vi "ProCoDA.vi"() -> ()   [LabVIEW 2015]
uses:
  Plant mode.ctl
  toolbar icons/open configuration.ctl
  toolbar icons/Save configuration.ctl
  toolbar icons/calibrator.ctl
  toolbar icons/edit rules.ctl
  switch and fraction.ctl
  toolbar icons/Data Source.ctl
  toolbar icons/file comment.ctl
  toolbar icons/log data.ctl
  TCP DAQ/Sensor data.ctl
  DAQ configuration/sensor cluster.ctl
  toolbar icons/peristaltic pump.ctl
  toolbar icons/help.ctl
  toolbar icons/Export pcm.ctl
  new config file.ctl
  calibration/Shared Data/share data boolean.ctl
  <vilib>/Utility/miscctls.llb/LVPositionTypeDef.ctl
  Plant state.ctl
  Distributed Daq/Data cmd.ctl
  DAQ configuration/Sensor buffer command.ctl
  file/file action.ctl
  Stamp/calibration commands.ctl
  default or user select.ctl
  calibration/Shared Data/share data command.ctl
  Calibration and Function folders.ctl
  <vilib>/Platform/browser.llb/Open URL in Default Browser (string).vi
panel:
  out "Legend:Position":T1
  in  "Swap Instance":T2
  in  "Name":string
  in  "Quit":bool
  out "auto datalogref":refnum<file>
  out "user datalog ref":refnum<file>
  in  "Tab Control":T3(tab)=enum."Process Operation"
  in  "Share data":T4
  in  "Datalog directory path":path
  in  "Auto data log interval":dbl=60.0 min=1.0 step=1.0
  out "Data Source":string
  in  "export pcm":T5
  out "sensor range error":bool
  out "Daq failure":bool
  in  "Peristaltic Pump":T6
  in  "Data Source":T7 caption="OK Button"
  out "data rate (Hz)":dbl
  out "Datalog File Failure":bool
  in  "Calibrate Sensors":T8
  in  "Edit Rules":T9
  in  "Save":T10
  in  "open":T11
  in  "Help Button":T12
  in  "File Comment":T13
  in  "Log Data":T14
  in  "User Data log interval":dbl=5.0 min=0.002 step=0.002
  out "read error":bool
  in  "Scrollbar":i32(c297)
  out "output descriptions":string[][](array[string])
  out "controls":T15 {"fractional duty" format="%#_3g"}
  in  "Operator Selected State":u16(ring)=1 items=["OFF", "Run pump"]
  out "Elapsed time in current state":dbl format="%.2f"
  out "Process State":u16(ring)=1 items=["OFF", "Run pump"]
  in  "Mode of Operation":T16=enum."Automatic Operation"
  out "Variables":cluster{string, "value":dbl}[](array[cluster]) {"value" format="%#_2g"}
  in  "history length":i32=1000 min=1
  in  "graph update interval":sgl=1.0 min=0.0001 format="%.4f"
  in  "Clear graph":bool
  out "Sensor Data":T17 {"Sensor array"."scaled" format="%.2f"; "Sensor array"."voltage" format="%.4f"; "Time" format="%<%I:%M:%S%2u %p\n%m/%d/%Y>T"}
  out "state graph":cluster{dbl[], dbl[]}(graph)
  in  "data to plot":i32[](listbox)
  out "Sensor graph":cluster{dbl[], dbl[]}[](graph)
  # "Method files (sensors, rules, calibrations)"
  # "Pump calibration"
  # "Calibrate the Analog Out"
  # "NI Input/Output device"
  # "Sensor configuration and calibration\nMeasure pH, D.O., Absorbance, etc."
  # "Data logging for experiments that span multiple days or if you need a state log."
  # "Control: states, rules, setpoints\nProgram the logic"
  # "Share data with or acquire data from other ProCoDA instances"
  # "Use this datalog method if you don't require a state log"
  # "s"
  # "0"
  # "1"
  # "2"
  # "3"
  # "4"
  # "5"
  # "6"
  # "7"
  # "pump off/on"
  # "0"
  # "pump cw/ccw"
  # "pump speed"
  # "pump off/on"
  # "1"
  # "pump cw/ccw"
  # "pump speed"
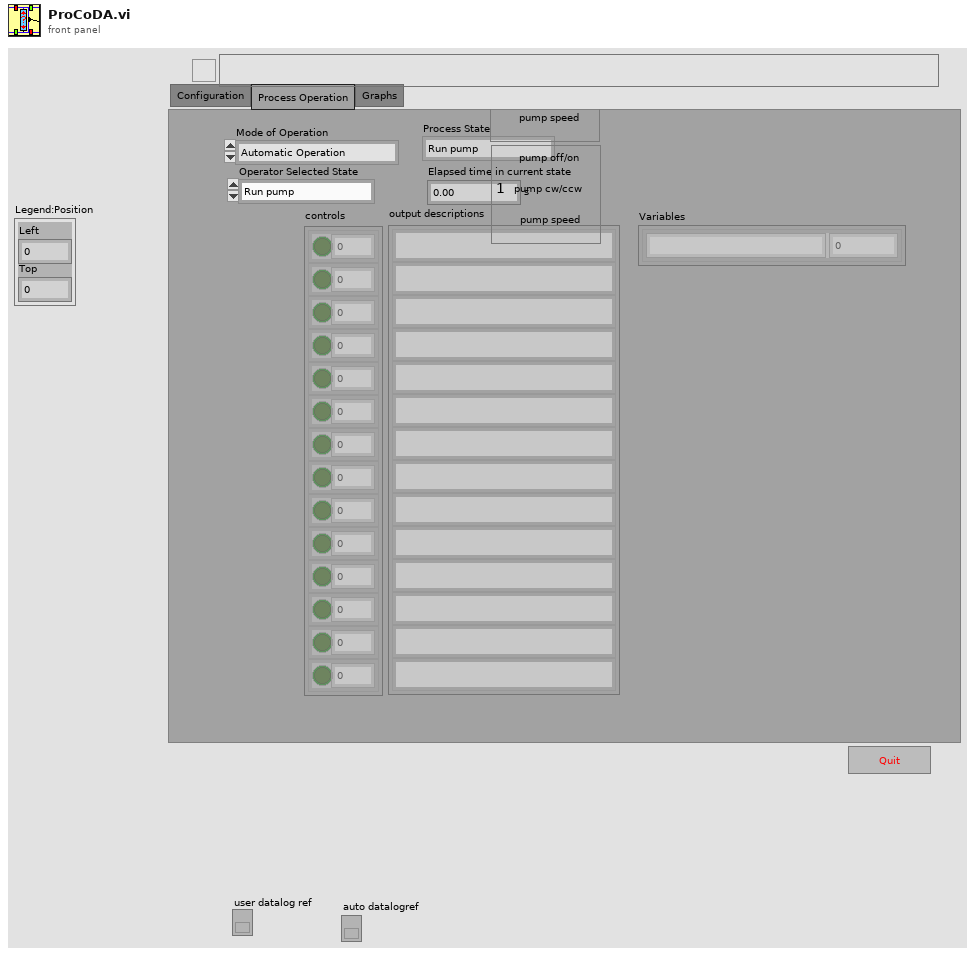
[diagram p1: front panel]
types:
  T1 = typedef "LVPositionTypeDef.ctl" = cluster{"Left":i32, "Top":i32}
  T2 = typedef "new config file.ctl" = bool
  T3 = enum32{"Configuration", "Process Operation", "Graphs"}
  T4 = typedef "share data boolean.ctl" = bool
  T5 = typedef "Export pcm.ctl" = bool
  T6 = typedef "peristaltic pump.ctl" = bool
  T7 = typedef "Data Source.ctl" = bool
  T8 = typedef "calibrator.ctl" = bool
  T9 = typedef "edit rules.ctl" = bool
  T10 = typedef "Save configuration.ctl" = bool
  T11 = typedef "open configuration.ctl" = bool
  T12 = typedef "help.ctl" = bool
  T13 = typedef "file comment.ctl" = bool
  T14 = typedef "log data.ctl" = bool
  T15 = typedef "switch and fraction.ctl" = cluster{"switch":bool, "fractional duty":dbl}[]
  T16 = typedef "Plant mode.ctl" = enum16{"Manual Locked in State", "Automatic Operation"}
  T17 = typedef "Sensor data.ctl" = cluster{" Sensor array":T18[], "Time":dbl}
  T18 = typedef "sensor cluster.ctl" = cluster{"voltage":sgl, "scaled":sgl, "units":string, "Out of Range":bool}
  T19 = typedef "file action.ctl" = enum16{"Save", "Open"}
  T20 = typedef "Sensor buffer command.ctl" = enum16{"read average", "read recent", "read all", "write", "set buffer size", "Read channel config", "Write channel config", "clear"}
  T21 = typedef "Data cmd.ctl" = enum16{"User config", "Ini config", "Read Data", "Close"}
  T22 = typedef "calibration commands.ctl" = enum16{"Get ini Path", "Save default values", "Save new calibration", "Read calibration", "Apply calibration", "Read STAMP mb", "Write STAMP mb"}
  T23 = typedef "share data command.ctl" = enum16{"Initialize from ini", "Update ini", "Write data", "Read data", "List my data", "List shared data", "Close"}
  T24 = typedef "default or user select.ctl" = enum16{"Default", "User select"}
  T25 = enum32{"invalid app kind", "Development System", "Run Time System", "Student Edition", "Embedded LabVIEW", "Evaluation", "Custom"}
  T26 = typedef "Calibration and Function folders.ctl" = enum16{"Sensors", "Functions", "Config File", "PublicAppFolder", "New ini File", "Set Config File", "Delete ini File"}
  T27 = enum16{"open", "open or create", "create or replace", "create", "open (read only)"}
  T28 = typedef "Plant state.ctl" = u16
  T29 = typedef "calibration values.ctl" = cluster{"target 1":dbl[unit], "target 2":dbl[unit], "measured 1":dbl[unit], "measured 2":dbl[unit]}
  T30 = typedef "write data cluster.ctl" = cluster{"Data interval (s)":sgl, "Shared Folder":path, "Write":bool[]}
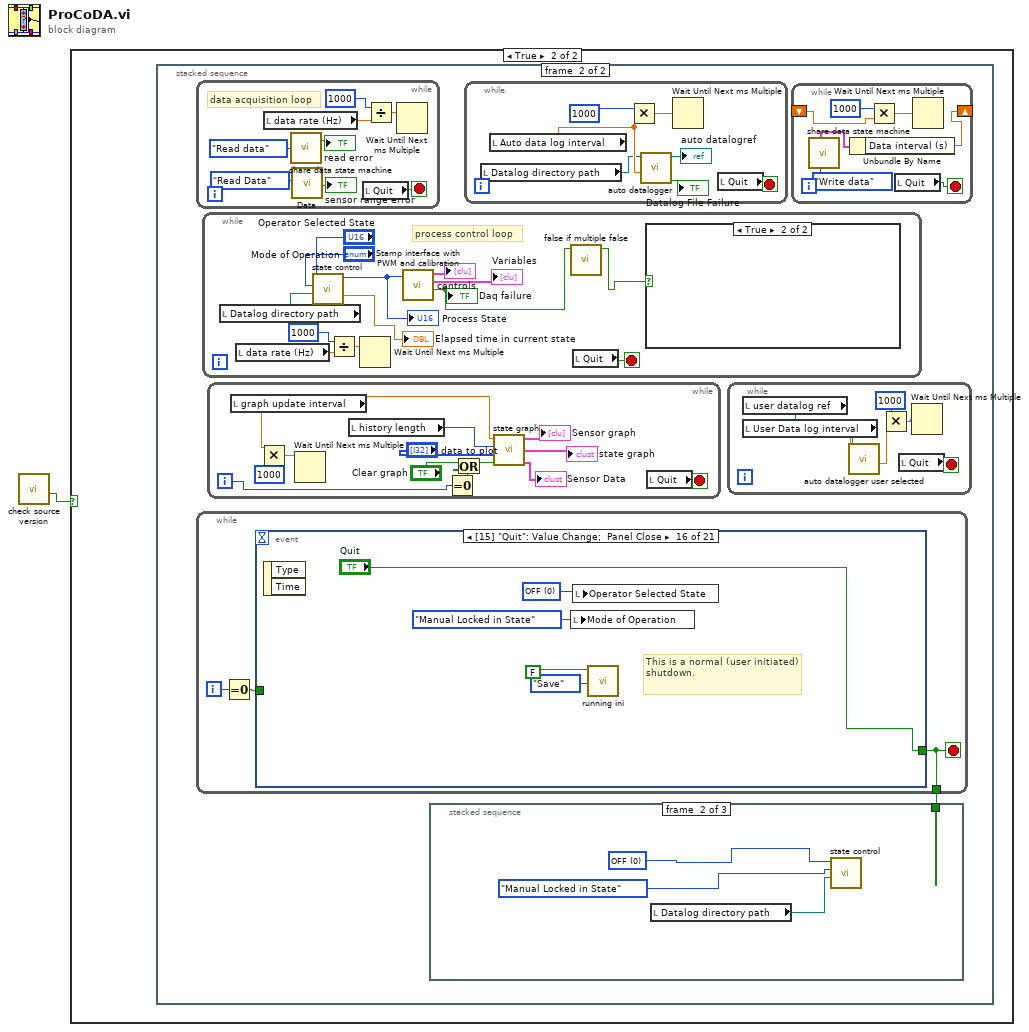
[diagram p0: block diagram]
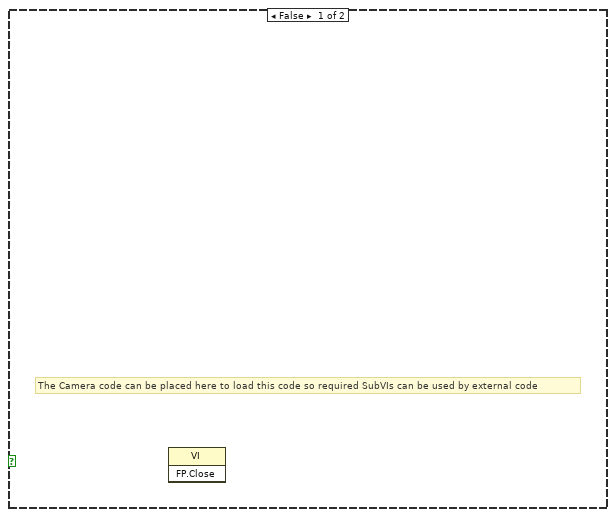
[diagram p2: hidden frame]
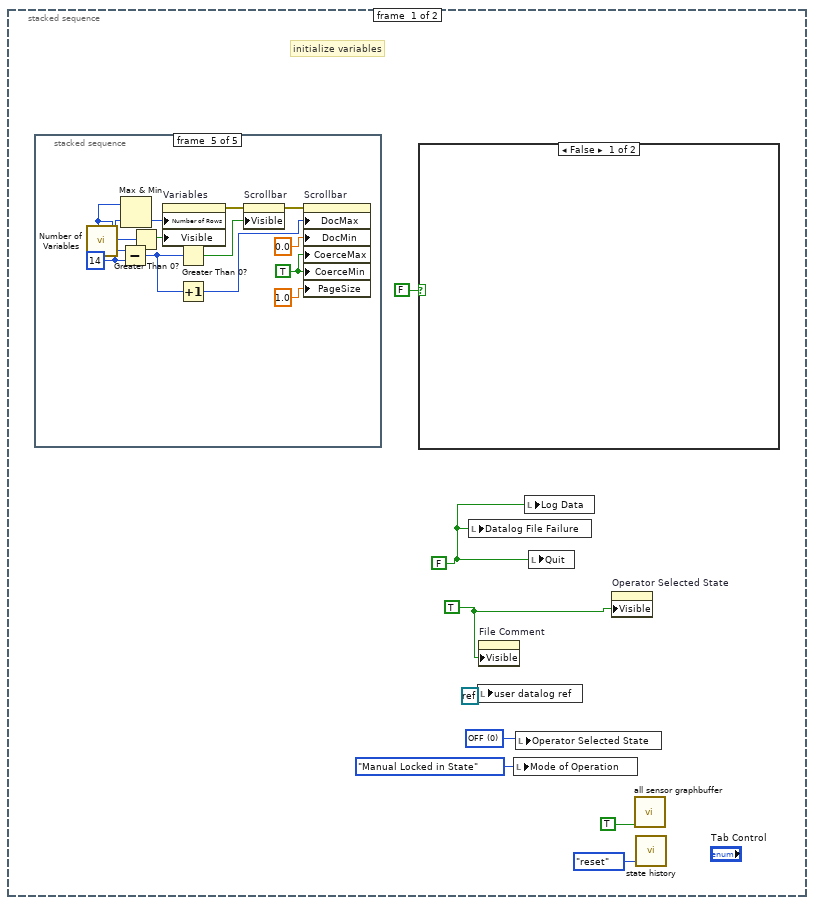
[diagram p3: hidden frame]
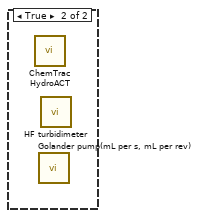
[diagram p4: hidden frame]
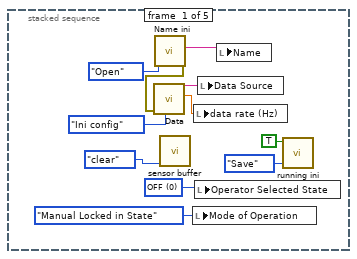
[diagram p5: hidden frame]
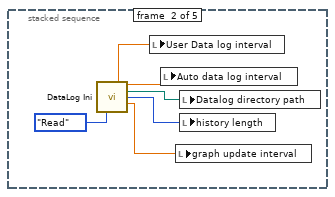
[diagram p6: hidden frame]
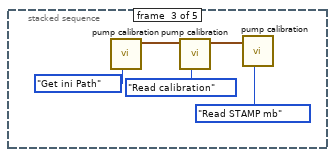
[diagram p7: hidden frame]
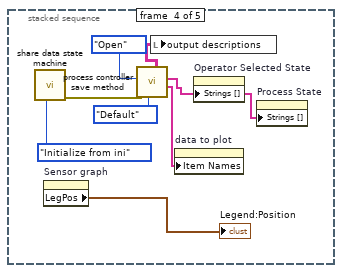
[diagram p8: hidden frame]
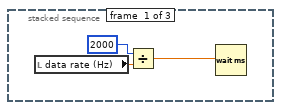
[diagram p9: hidden frame]
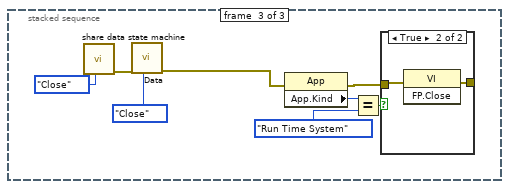
[diagram p10: hidden frame]
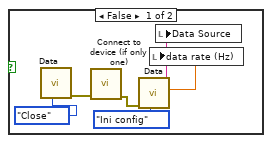
[diagram p12: hidden frame]
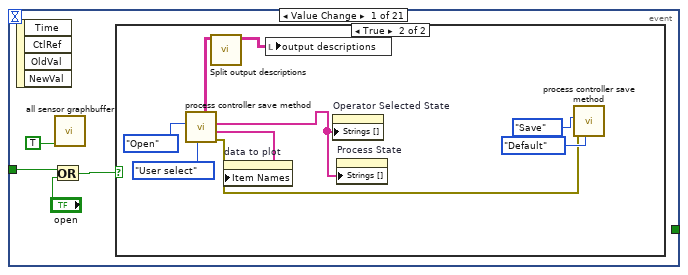
[diagram p13: hidden frame]
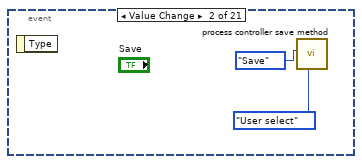
[diagram p15: hidden frame]
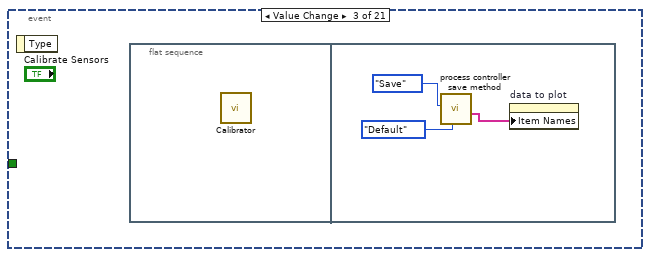
[diagram p16: hidden frame]
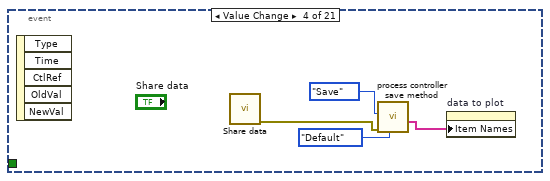
[diagram p17: hidden frame]
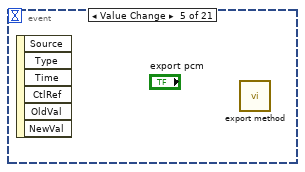
[diagram p18: hidden frame]
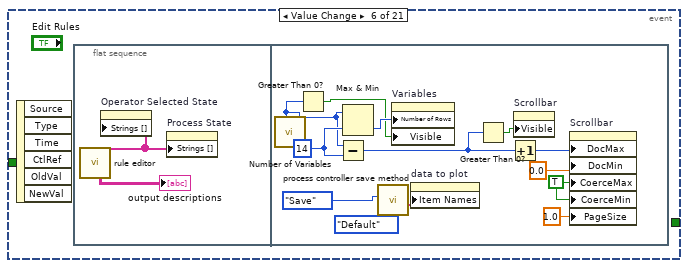
[diagram p19: hidden frame]
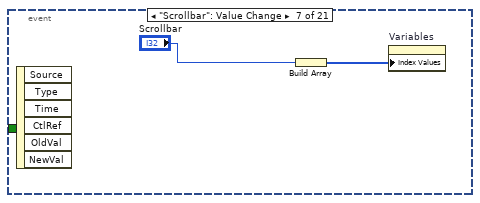
[diagram p20: hidden frame]
diagram:
  n1 = call "check source version.vi"() -> ("continue running?"=w1:bool)  [unwired: 5 in, 2 out]
  n2 = case shown="True" w1 {
    frame False {
      # "The Camera code can be placed here to load this code so required SubVIs can be used by external code"
      n3 = invoke class="VI" method="FP.Close"() -> ()  [unwired: 3 in, 3 out]
    }
    frame True {
      n4 = stacked-sequence {
        frame #0 {
          w6 = T28 0 items=["OFF"] ("Operator Selected State")
          w4 = TRUE ("stop")
          w3 = FALSE ("stop")
          # "initialize variables"
          n5 = stacked-sequence {
            frame #0 {
              w12 = T28 0 items=["OFF"] ("Operator Selected State")
              n6 = call "Name ini.vi"("Action"=file_action."Open") -> ("error out"=w10:errorcluster, "Name out"=w16:string)  [unwired: 7 in]
              n7 = call "Data.vi"("Data Command"=Data_cmd."Ini config", "error in"=w10) -> ("data rate (Hz)"=w20:dbl, "Daq Name"=w18:string)  [unwired: 6 in, 2 out]
              n8 = call "sensor buffer.vi"("command"=Sensor_buffer_command."clear") -> ()  [unwired: 6 in, 5 out]
              n9 = local write "Mode of Operation"(Plant_mode."Manual Locked in State" ("Mode of Operation")) -> ()
              n10 = local write "data rate (Hz)"(w20) -> ()
              n11 = local write "Operator Selected State"(w12) -> ()
              n12 = local write "Data Source"(w18) -> ()
              n13 = local write "Name"(w16) -> ()
              n14 = call "running ini.vi"("running in"=TRUE ("running"), "Action"=file_action."Save") -> ()  [unwired: 4 in, 1 out]
            }
            frame #1 {
              n15 = call "DataLog Ini.vi"("Ini Cmd"=enum16{"Read", "Write"}."Read") -> ("User Data log interval out"=w26:dbl, "Auto data log interval out"=w22:dbl, "Datalog directory path out"=w23:path, "history length out"=w24:i32, "graph update interval out"=w25:dbl)  [unwired: 9 in, 1 out]
              n16 = local write "User Data log interval"(w26) -> ()
              n17 = local write "Auto data log interval"(w22) -> ()
              n18 = local write "graph update interval"(w25) -> ()
              n19 = local write "Datalog directory path"(w23) -> ()
              n20 = local write "history length"(w24) -> ()
            }
            frame #2 {
              n21 = call "pump calibration.vi"("pump cal command"=calibration_commands."Get ini Path") -> ("Pump Calibration out"=w28:T29)  [unwired: 7 in, 3 out]
              n22 = call "pump calibration.vi"("pump cal command"=calibration_commands."Read calibration", "Pump Calibration in"=w28) -> ("Pump Calibration out"=w31:T29)  [unwired: 6 in, 3 out]
              n23 = call "pump calibration.vi"("pump cal command"=calibration_commands."Read STAMP mb", "Pump Calibration in"=w31) -> ()  [unwired: 6 in, 4 out]
            }
            frame #3 {
              n24 = call "share data state machine.vi"("Share data command"=share_data_command."Initialize from ini") -> ("error out"=w34:errorcluster)  [unwired: 4 in, 6 out]
              n25 = property on="Sensor graph" class="XYGraph (strict)"() -> ("LegPos"=→"Legend:Position":T1)  [unwired: 2 in, 2 out]
              n26 = call "process controller save method.vi"("default or user"=default_or_user_select."Default", "error in (not an error)"=w34, "Action"=file_action."Open") -> ("sensor &var names"=w35:string[], "State names"=w37:string[], "output descriptions out"=w36:string[][])  [unwired: 5 in, 1 out]
              n27 = local write "output descriptions"(w36) -> ()
              n28 = property on="data to plot" class="LstBox (strict)"("Item Names"=w35) -> ()  [unwired: 2 in, 2 out]
              n29 = property on="Operator Selected State" class="Ring (strict)"("Strings []"=w37) -> ()  [unwired: 2 in, 2 out]
              n30 = property on="Process State" class="Ring (strict)"("Strings []"=w37) -> ()  [unwired: 2 in, 2 out]
            }
            frame #4 {
              w47 = TRUE ("Coerce Maximum Value")
              w49 = 14 ("y")
              n31 = call "Number of Variables.vi"() -> ("Number of Variables"=w40:i32)  [unwired: 11 in]
              n32 = Subtract(x=w40, y=w49) -> (x-y=w42:i32)
              n33 = Max & Min(x=w40, y=w49) -> (min(x,y)=w43:i32)  [unwired: 1 out]
              n34 = Greater Than 0?(x=w40) -> (x > 0?=w41:bool)
              n35 = property on="Variables" class="Arr (strict)"("Number of Rows"=w43, "Visible"=w41) -> (error out=w50:errorcluster)  [unwired: 2 in, 1 out]
              n36 = Greater Than 0?(x=w42) -> (x > 0?=w44:bool)
              n37 = Increment(x=w42) -> (x+1=w45:i32)
              n38 = property on="Scrollbar" class="Scroll (strict)"(error in=w50, "Visible"=w44) -> (error out=w51:errorcluster)  [unwired: 1 in, 1 out]
              n39 = property on="Scrollbar" class="Scroll (strict)"(error in=w51, "DocMax"=w45, "DocMin"=0.0 ("Doc Min"), "CoerceMax"=w47, "CoerceMin"=w47, "PageSize"=1.0 ("Page Size")) -> ()  [unwired: 1 in, 2 out]
            }
          }
          n40 = case shown="False" FALSE {
            frame False {
            }
            frame True {
              n41 = call "ChemTrac HydroACT.vi"() -> ()  [unwired: 6 in, 2 out]
              n42 = call "Golander pump(mL per s, mL per rev).vi"() -> ()  [unwired: 6 in, 2 out]
              n43 = call "HF turbidimeter.vi"() -> ()  [unwired: 6 in, 2 out]
            }
          }
          n44 = local write "Datalog File Failure"(w3) -> ()
          n45 = local write "user datalog ref"(refnum<k0> refnum) -> ()
          n46 = property on="File Comment" class="Bool"("Visible"=w4) -> ()  [unwired: 2 in, 2 out]
          n47 = local write "Mode of Operation"(Plant_mode."Manual Locked in State" ("Mode of Operation")) -> ()
          n48 = local write "Operator Selected State"(w6) -> ()
          n49 = local write "Log Data"(w3) -> ()
          n50 = local write "Quit"(w3) -> ()
          n51 = property on="Operator Selected State" class="Ring (strict)"("Visible"=w4) -> ()  [unwired: 2 in, 2 out]
          n52 = call "all sensor graphbuffer.vi"("Reset"=TRUE) -> ()  [unwired: 8 in, 3 out]
          n53 = call "state history.vi"("command"=enum16{"write", "read", "reset"}."reset") -> ()  [unwired: 2 in, 1 out]
        }
        frame #1 {
          n54 = while {
            stop <- w128 stop-if-true
            # "data acquisition loop"
            n55 = local read "data rate (Hz)"() -> (w123:dbl)
            n56 = call "share data state machine.vi"("Share data command"=share_data_command."Read data") -> ("read error"=→"read error":bool)  [unwired: 4 in, 6 out]
            n57 = call "Data.vi"("Data Command"=Data_cmd."Read Data") -> ("Range error"=→"sensor range error":bool)  [unwired: 7 in, 3 out]
            n58 = local read "Quit"() -> (w128:bool)
            n59 = Divide(x=1000, y=w123) -> (x/y=w121:dbl)
            n60 = Wait Until Next ms Multiple(millisecond multiple=w121) -> ()  [unwired: 1 out]
          }
          n61 = while {
            tunnel: [w129] -> w52
            i -> [w130]
            stop <- w129 stop-if-true
            n62 = Equal To 0?(x=w130) -> (x = 0?=w131:bool)
            n63 = event shown="[15] \"Quit\": Value Change;  Panel Close" {
              selector: _ -> [_ _ _ _ _ _ _ _ _ _ _ _ _ _ _ _ _ _ _ _ _]
              dyn-events: _ -> [_ _ _ _ _ _ _ _ _ _ _ _ _ _ _ _ _ _ _ _ _]
              timeout: _ -> [_ _ _ _ _ _ _ _ _ _ _ _ _ _ _ _ _ _ _ _ _]
              tunnel: w131 -> [w133 _ _ _ _ _ _ _ _ _ _ _ _ _ _ _ _ _ _ _ _]
              tunnel: [_ _ _ _ _ _ _ _ _ _ _ _ _ _ _ "Quit" w216 w219 _ _ _] -> w129
              event Value Change {
                n64 = event-data() -> ()  [unwired: 1 in, 4 out]
                n65 = Or(x=w133, y="open") -> (x .or. y?=w132:T11)
                n66 = call "all sensor graphbuffer.vi"("Reset"=TRUE) -> ()  [unwired: 8 in, 3 out]
                n67 = case shown="True" w132 {
                  frame False {
                  }
                  frame True {
                    n68 = call "process controller save method.vi"("default or user"=default_or_user_select."User select", "Action"=file_action."Open") -> ("error out"=w136:errorcluster, "sensor &var names"=w143:string[], "State names"=w142:string[], "output descriptions out"=w138:string[][])  [unwired: 6 in]
                    n69 = call "Split output descriptions.vi"("output descriptions combined"=w138) -> ("output descriptions"=w137:string[][])  [unwired: 9 in, 1 out]
                    n70 = property on="data to plot" class="LstBox (strict)"("Item Names"=w143) -> ()  [unwired: 2 in, 2 out]
                    n71 = local write "output descriptions"(w137) -> ()
                    n72 = property on="Operator Selected State" class="Ring (strict)"("Strings []"=w142) -> ()  [unwired: 2 in, 2 out]
                    n73 = property on="Process State" class="Ring (strict)"("Strings []"=w142) -> ()  [unwired: 2 in, 2 out]
                    n74 = call "process controller save method.vi"("default or user"=default_or_user_select."Default", "error in (not an error)"=w136, "Action"=file_action."Save") -> ()  [unwired: 5 in, 4 out]
                  }
                }
              }
              event Value Change {
                n75 = event-data() -> ()  [unwired: 1 in, 1 out]
                n76 = call "process controller save method.vi"("default or user"=default_or_user_select."User select", "Action"=file_action."Save") -> ()  [unwired: 6 in, 4 out]
              }
              event Value Change {
                n77 = event-data() -> ()  [unwired: 1 in, 1 out]
                n78 = flat-sequence {
                  frame #0 {
                    n79 = call "Calibrator.vi"() -> ()  [unwired: 9 in, 2 out]
                  }
                  frame #1 {
                    n80 = call "process controller save method.vi"("default or user"=default_or_user_select."Default", "Action"=file_action."Save") -> ("sensor &var names"=w147:string[])  [unwired: 6 in, 3 out]
                    n81 = property on="data to plot" class="LstBox (strict)"("Item Names"=w147) -> ()  [unwired: 2 in, 2 out]
                  }
                }
              }
              event Value Change {
                n82 = event-data() -> ()  [unwired: 1 in, 5 out]
                n83 = call "Share data.vi"() -> ("error out"=w150:errorcluster)  [unwired: 11 in]
                n84 = call "process controller save method.vi"("default or user"=default_or_user_select."Default", "error in (not an error)"=w150, "Action"=file_action."Save") -> ("sensor &var names"=w151:string[])  [unwired: 5 in, 3 out]
                n85 = property on="data to plot" class="LstBox (strict)"("Item Names"=w151) -> ()  [unwired: 2 in, 2 out]
              }
              event Value Change {
                n86 = event-data() -> ()  [unwired: 1 in, 6 out]
                n87 = call "export method.vi"() -> ()  [unwired: 1 in]
              }
              event Value Change {
                n88 = event-data() -> ()  [unwired: 1 in, 6 out]
                n89 = flat-sequence {
                  frame #0 {
                    n90 = call "rule editor.vi"() -> ("output descriptions out"=→"output descriptions":string[][], "State names"=w154:string[])  [unwired: 8 in, 2 out]
                    n91 = property on="Operator Selected State" class="Ring (strict)"("Strings []"=w154) -> ()  [unwired: 2 in, 2 out]
                    n92 = property on="Process State" class="Ring (strict)"("Strings []"=w154) -> ()  [unwired: 2 in, 2 out]
                  }
                  frame #1 {
                    w159 = TRUE ("Coerce Maximum Value")
                    w163 = 14 ("y")
                    n93 = call "Number of Variables.vi"() -> ("Number of Variables"=w157:i32)  [unwired: 11 in]
                    n94 = Greater Than 0?(x=w157) -> (x > 0?=w156:bool)
                    n95 = Subtract(x=w157, y=w163) -> (x-y=w162:i32)
                    n96 = Max & Min(x=w157, y=w163) -> (min(x,y)=w165:i32)  [unwired: 1 out]
                    n97 = call "process controller save method.vi"("default or user"=default_or_user_select."Default", "Action"=file_action."Save") -> ("sensor &var names"=w167:string[])  [unwired: 6 in, 3 out]
                    n98 = property on="Variables" class="Arr (strict)"("Number of Rows"=w165, "Visible"=w156) -> ()  [unwired: 2 in, 2 out]
                    n99 = property on="data to plot" class="LstBox (strict)"("Item Names"=w167) -> ()  [unwired: 2 in, 2 out]
                    n100 = Greater Than 0?(x=w162) -> (x > 0?=w161:bool)
                    n101 = Increment(x=w162) -> (x+1=w160:i32)
                    n102 = property on="Scrollbar" class="Scroll (strict)"("Visible"=w161) -> ()  [unwired: 2 in, 2 out]
                    n103 = property on="Scrollbar" class="Scroll (strict)"("DocMax"=w160, "DocMin"=0.0 ("Doc Min"), "CoerceMax"=w159, "CoerceMin"=w159, "PageSize"=1.0 ("Page Size")) -> ()  [unwired: 2 in, 2 out]
                  }
                }
              }
              event "Scrollbar": Value Change {
                n104 = event-data() -> ()  [unwired: 1 in, 6 out]
                n105 = Build Array("Scrollbar") -> (w169:i32[])
                n106 = property on="Variables" class="Arr (strict)"("Index Values"=w169) -> ()  [unwired: 2 in, 2 out]
              }
              event Value Change {
                n107 = event-data() -> ()  [unwired: 1 in, 6 out]
                n108 = local read "user datalog ref"() -> (w172:refnum<file>)
                n109 = local read "auto datalogref"() -> (w171:refnum<file>)
                n110 = Not A Number/Path/Refnum?(number/path/refnum=w172) -> (NaN/Path/Refnum?=w174:bool)
                n111 = Select(t=w171, s=w174, f=w172) -> (s? t:f=w173:refnum<file>)
                n112 = call "Write comment to file.vi"("refnum"=w173) -> ()  [unwired: 7 in, 2 out]
              }
              event Value Change {
                n113 = event-data() -> ()  [unwired: 1 in, 6 out]
                n114 = case shown="True" "Log Data" {
                  tunnel: [refnum<k0> refnum w183] -> w176
                  frame False {
                    n115 = local read "user datalog ref"() -> (w178:refnum<file>)
                    n116 = Close File(refnum=w178) -> ()  [unwired: 1 in, 2 out]
                  }
                  frame True {
                    n117 = call "Calibration and Function folders.vi"("Folder"=Calibration_and_Function_folders."PublicAppFolder") -> ("Selected Folder"=w179:path)  [unwired: 9 in, 1 out]
                    n118 = call <vilib>:"Open_Create_Replace File.vi"("pattern"="*.tsv", "default name"="New Datalog file", "prompt"="Create a new datalog file", "function (open:0)"=T27."open or create", "start path  (Not A Path)"=w179) -> ("error out"=w181:errorcluster, "refnum"=w183:refnum<file>)  [unwired: 3 in, 2 out]
                    n119 = case shown="Error" w181 {
                      frame No Error {
                      }
                      frame Error {
                        n120 = local write "Log Data"(T14 FALSE ("Log Data")) -> ()
                      }
                    }
                  }
                }
                "user datalog ref" <- w176
              }
              event Value Change {
                n121 = event-data() -> ()  [unwired: 1 in, 6 out]
                n122 = call "Data.vi"("Data Command"=Data_cmd."User config") -> ("data rate (Hz)"=→"data rate (Hz)":dbl, "Daq Name"=→"Data Source":string)  [unwired: 7 in, 2 out]
              }
              event Value Change {
                n123 = event-data() -> ()  [unwired: 1 in, 6 out]
                n124 = call-poly <vilib>:"Open URL in Default Browser.vi"("URL"="https://monroews.github.io/EnvEngLabTextbook/ProCoDA/ProCoDA.html#procoda-process-control-and-data-acquisition") -> ()  [unwired: 5 in, 2 out]
              }
              event "Clear graph": Value Change {
                n125 = event-data() -> ()  [unwired: 1 in, 5 out]
                n126 = call "state history.vi"("command"=enum16{"write", "read", "reset"}."reset") -> ()  [unwired: 2 in, 1 out]
              }
              event "data to plot": Value Change; "data to plot": Mouse Down {
                n127 = event-data() -> ()  [unwired: 1 in, 3 out]
                n128 = local read "data to plot"() -> (w196:i32[])
                n129 = property on="data to plot" class="LstBox (strict)"() -> ("Item Names"=w197:string[])  [unwired: 2 in, 2 out]
                n130 = for {
                  tunnel: w197 -> [w203]
                  tunnel: w196 -> [w204] mode=indexing
                  tunnel: [w201] -> w194
                  i -> [w201]
                  n131 = Index Array(array=w203, index=w204) -> (element=w202:string)
                  n132 = property on="Sensor graph" class="XYGraph (strict)"("Active Plot"=w201, "Plot.Plot Name"=w202, "ActYScl"=w201) -> ()  [unwired: 2 in, 2 out]
                }
                n133 = Index Array(array=w196, index=0) -> (element=w199:i32)
                n134 = Build Array(w199) -> (w200:i32[])
                n135 = property on="Sensor array" class="Arr (strict)"("Index Values"=w200) -> ()  [unwired: 2 in, 2 out]
                n136 = local read "Legend:Position"() -> (w195:T1)
                n137 = Increment(x=w194) -> (x+1=w193:i32)
                n138 = property on="Sensor graph" class="XYGraph (strict)"("LegNumRows"=w193, "LegPos"=w195) -> ()  [unwired: 2 in, 2 out]
              }
              event "Datalog directory path", "Auto data log interval", "graph update interval", "history length", "User Data log interval": Value Change {
                n139 = event-data() -> ()  [unwired: 1 in, 6 out]
                n140 = call "DataLog Ini.vi"("Auto data log interval"="Auto data log interval", "User Data log interval"="User Data log interval", "Datalog directory path"="Datalog directory path", "history length"="history length", "graph update interval"="graph update interval", "Ini Cmd"=enum16{"Read", "Write"}."Write") -> ()  [unwired: 4 in, 6 out]
              }
              event Value Change {
                n141 = event-data() -> ()  [unwired: 1 in, 6 out]
                n142 = call "pump calibration dialog.vi"() -> ()  [unwired: 1 in]
              }
              event "Quit": Value Change; Panel Close {
                w211 = T28 0 items=["OFF"] ("Operator Selected State")
                (unwired) TRUE ("Quit")
                # "This is a normal (user initiated) shutdown."
                n143 = event-data() -> ()  [unwired: 1 in, 2 out]
                n144 = local write "Mode of Operation"(Plant_mode."Manual Locked in State" ("Mode of Operation")) -> ()
                n145 = local write "Operator Selected State"(w211) -> ()
                n146 = call "running ini.vi"("running in"=FALSE ("running"), "Action"=file_action."Save") -> ()  [unwired: 4 in, 1 out]
              }
              event Panel Close? {
                w216 = TRUE ("Quit")
                # "This is a normal (user initiated) shutdown."
                n147 = event-data() -> ()  [unwired: 1 in, 4 out]
                n148 = call "running ini.vi"("running in"=FALSE ("running"), "Action"=file_action."Save") -> ()  [unwired: 4 in, 1 out]
                n149 = local write "Quit"(w216) -> ()
                n150 = event-data("Discard?"=w216) -> ()  [unwired: 1 in, 1 out]
              }
              event Application Instance Close? {
                w219 = TRUE ("Quit")
                n151 = event-data() -> ()  [unwired: 1 in, 5 out]
                n152 = local write "Quit"(w219) -> ()
                n153 = event-data("Discard?"=w219) -> ()  [unwired: 2 in, 1 out]
              }
              event "Operator Selected State": Value Change; "Operator Selected State": Mouse Up {
                n154 = event-data() -> ()  [unwired: 1 in, 3 out]
                n155 = local read "Operator Selected State"() -> (w221:u16)
                n156 = local read "Datalog directory path"() -> (w220:path)
                n157 = call "state control.vi"("Datalog directory path"=w220, "Plant Mode of Operation"=Plant_mode."Manual Locked in State", "Operator Selected State"=w221) -> ()  [unwired: 6 in, 3 out]
              }
              event Value Change {
                n158 = event-data() -> ()  [unwired: 1 in, 5 out]
                n159 = call "Select ini file.vi"() -> ("error out"=w223:errorcluster, "Name"=w224:string)  [unwired: 9 in]
                n160 = local write "Name"(w224) -> ()
                n161 = stacked-sequence {
                  tunnel: w223 -> [_ _ _ _ _ _]
                  frame #0 {
                    n162 = call "share data state machine.vi"("Share data command"=share_data_command."Initialize from ini") -> ("error out"=w228:errorcluster)  [unwired: 4 in, 6 out]
                    n163 = call "process controller save method.vi"("default or user"=default_or_user_select."Default", "error in (not an error)"=w228, "Action"=file_action."Open") -> ("sensor &var names"=w227:string[], "State names"=w226:string[], "output descriptions out"=w225:string[][])  [unwired: 5 in, 1 out]
                    n164 = local write "output descriptions"(w225) -> ()
                    n165 = property on="data to plot" class="LstBox (strict)"("Item Names"=w227) -> ()  [unwired: 2 in, 2 out]
                    n166 = property on="Operator Selected State" class="Ring (strict)"("Strings []"=w226) -> ()  [unwired: 2 in, 2 out]
                    n167 = property on="Process State" class="Ring (strict)"("Strings []"=w226) -> ()  [unwired: 2 in, 2 out]
                  }
                  frame #1 {
                    w235 = T28 0 items=["OFF"] ("Operator Selected State")
                    n168 = call "Data.vi"("Data Command"=Data_cmd."Close") -> ("error out"=w232:errorcluster)  [unwired: 7 in, 3 out]
                    n169 = call "sensor buffer.vi"("command"=Sensor_buffer_command."clear") -> ()  [unwired: 6 in, 5 out]
                    n170 = call "Data.vi"("Data Command"=Data_cmd."Ini config", "error in"=w232) -> ("data rate (Hz)"=w243:dbl, "Daq Name"=w241:string)  [unwired: 6 in, 2 out]
                    n171 = local write "Operator Selected State"(w235) -> ()
                    n172 = call "Name ini.vi"("Action"=file_action."Open") -> ("Name out"=w239:string)  [unwired: 7 in, 1 out]
                    n173 = local write "Mode of Operation"(Plant_mode."Manual Locked in State" ("Mode of Operation")) -> ()
                    n174 = local write "data rate (Hz)"(w243) -> ()
                    n175 = local write "Data Source"(w241) -> ()
                    n176 = local write "Name"(w239) -> ()
                    n177 = call "running ini.vi"("running in"=TRUE ("running"), "Action"=file_action."Save") -> ()  [unwired: 4 in, 1 out]
                  }
                  frame #2 {
                    n178 = call "DataLog Ini.vi"("Ini Cmd"=enum16{"Read", "Write"}."Read") -> ("User Data log interval out"=w249:dbl, "Auto data log interval out"=w245:dbl, "Datalog directory path out"=w246:path, "history length out"=w247:i32, "graph update interval out"=w248:dbl)  [unwired: 9 in, 1 out]
                    n179 = local write "User Data log interval"(w249) -> ()
                    n180 = local write "Auto data log interval"(w245) -> ()
                    n181 = local write "graph update interval"(w248) -> ()
                    n182 = local write "Datalog directory path"(w246) -> ()
                    n183 = local write "history length"(w247) -> ()
                  }
                  frame #3 {
                    n184 = call "pump calibration.vi"("pump cal command"=calibration_commands."Get ini Path") -> ("Pump Calibration out"=w251:T29)  [unwired: 7 in, 3 out]
                    n185 = call "pump calibration.vi"("pump cal command"=calibration_commands."Read calibration", "Pump Calibration in"=w251) -> ("Pump Calibration out"=w254:T29)  [unwired: 6 in, 3 out]
                    n186 = call "pump calibration.vi"("pump cal command"=calibration_commands."Read STAMP mb", "Pump Calibration in"=w254) -> ()  [unwired: 6 in, 4 out]
                  }
                  frame #4 {
                    w263 = TRUE ("Coerce Maximum Value")
                    w265 = 14 ("y")
                    n187 = Wait (ms)(milliseconds to wait=u32 1000) -> ()  [unwired: 1 out]
                    n188 = call "Number of Variables.vi"() -> ("Number of Variables"=w256:i32)  [unwired: 11 in]
                    n189 = Subtract(x=w256, y=w265) -> (x-y=w258:i32)
                    n190 = Max & Min(x=w256, y=w265) -> (min(x,y)=w259:i32)  [unwired: 1 out]
                    n191 = Greater Than 0?(x=w256) -> (x > 0?=w257:bool)
                    n192 = property on="Variables" class="Arr (strict)"("Number of Rows"=w259, "Visible"=w257) -> (error out=w266:errorcluster)  [unwired: 2 in, 1 out]
                    n193 = Greater Than 0?(x=w258) -> (x > 0?=w260:bool)
                    n194 = Increment(x=w258) -> (x+1=w261:i32)
                    n195 = property on="Scrollbar" class="Scroll (strict)"(error in=w266, "Visible"=w260) -> (error out=w267:errorcluster)  [unwired: 1 in, 1 out]
                    n196 = property on="Scrollbar" class="Scroll (strict)"(error in=w267, "DocMax"=w261, "DocMin"=0.0 ("Doc Min"), "CoerceMax"=w263, "CoerceMin"=w263, "PageSize"=1.0 ("Page Size")) -> ()  [unwired: 1 in, 2 out]
                  }
                  frame #5 {
                    n197 = call "process controller save method.vi"("default or user"=default_or_user_select."Default", "Action"=file_action."Save") -> ("sensor &var names"=w270:string[])  [unwired: 6 in, 3 out]
                    n198 = property on="data to plot" class="LstBox (strict)"("Item Names"=w270) -> ()  [unwired: 2 in, 2 out]
                  }
                }
              }
              event "Name": Value Change {
                n199 = event-data() -> ()  [unwired: 1 in, 5 out]
                n200 = call "Name ini.vi"("Action"=file_action."Save", "Name in"="Name") -> ()  [unwired: 6 in, 2 out]
              }
            }
          }
          n201 = while {
            stop <- w102 stop-if-true
            # "process control loop"
            n202 = local read "Datalog directory path"() -> (w109:path)
            n203 = local read "data rate (Hz)"() -> (w103:dbl)
            n204 = call "state control.vi"("Datalog directory path"=w109, "Plant Mode of Operation"="Mode of Operation", "Operator Selected State"="Operator Selected State") -> ("Elapsed time in current state"=→"Elapsed time in current state":dbl, "Plant State out"=w111:u16)  [unwired: 6 in, 1 out]
            "Process State" <- w111
            n205 = Divide(x=1000, y=w103) -> (x/y=w105:dbl)
            n206 = Wait Until Next ms Multiple(millisecond multiple=w105) -> ()  [unwired: 1 out]
            n207 = call "Stamp interface with PWM and calibration.vi"("Plant State"=w111) -> ("NI board success"=w107:bool, "Variables"=→"Variables":cluster{string, "value":dbl}[], "Controls out 1"=→"controls":T15)  [unwired: 7 in, 1 out]
            "Daq failure" <- w107
            n208 = call "false if multiple false.vi"("Fail"=w107) -> ("Multiple fail"=w106:bool)  [unwired: 10 in]
            n209 = local read "Quit"() -> (w102:bool)
            n210 = case shown="True" w106 {
              frame False {
                n211 = call "Data.vi"("Data Command"=Data_cmd."Close") -> ("error out"=w116:errorcluster)  [unwired: 7 in, 3 out]
                n212 = call "Connect to device (if only one).vi"("error in"=w116) -> ("error out"=w117:errorcluster)  [unwired: 10 in]
                n213 = call "Data.vi"("Data Command"=Data_cmd."Ini config", "error in"=w117) -> ("data rate (Hz)"=w120:dbl, "Daq Name"=w119:string)  [unwired: 6 in, 2 out]
                n214 = local write "data rate (Hz)"(w120) -> ()
                n215 = local write "Data Source"(w119) -> ()
              }
              frame True {
              }
            }
          }
          n216 = while {
            i -> [w90]
            stop <- w99 stop-if-true
            n217 = local read "graph update interval"() -> (w94:sgl)
            n218 = Multiply(x=w94, y=i16 1000) -> (x*y=w100:sgl)
            n219 = Wait Until Next ms Multiple(millisecond multiple=w100) -> ()  [unwired: 1 out]
            n220 = local read "history length"() -> (w93:i32)
            n221 = Equal To 0?(x=w90) -> (x = 0?=w89:bool)
            n222 = Or(x="Clear graph", y=w89) -> (x .or. y?=w91:bool)
            n223 = call "state graph.vi"("Clear graph"=w91, "sensor to plot"="data to plot", "history length"=w93, "graph update interval"=w94) -> ("Sensor Data Smoothed"=→"Sensor Data":T17, "state graph"=→"state graph":cluster{dbl[], dbl[]}, "sensor graph array"=→"Sensor graph":cluster{dbl[], dbl[]}[])  [unwired: 1 in]
            n224 = local read "Quit"() -> (w99:bool)
          }
          n225 = stacked-sequence {
            tunnel: w52 -> [_ _ _]
            frame #0 {
              n226 = local read "data rate (Hz)"() -> (w62:dbl)
              n227 = Divide(x=2000, y=w62) -> (x/y=w60:dbl)
              n228 = Wait (ms)(milliseconds to wait=w60) -> ()  [unwired: 1 out]
            }
            frame #1 {
              w63 = T28 0 items=["OFF"] ("Operator Selected State")
              n229 = local read "Datalog directory path"() -> (w65:path)
              n230 = call "state control.vi"("Datalog directory path"=w65, "Plant Mode of Operation"=Plant_mode."Manual Locked in State" ("Mode of Operation"), "Operator Selected State"=w63) -> ()  [unwired: 6 in, 3 out]
            }
            frame #2 {
              n231 = call "share data state machine.vi"("Share data command"=share_data_command."Close") -> ("error out"=w66:errorcluster)  [unwired: 4 in, 6 out]
              n232 = call "Data.vi"("Data Command"=Data_cmd."Close", "error in"=w66) -> ("error out"=w68:errorcluster)  [unwired: 6 in, 3 out]
              n233 = property class="App"(error in=w68) -> (error out=w73:errorcluster, "App.Kind"=w71:T25)  [unwired: 1 in, 1 out]
              n234 = Equal?(x=w71, y=T25."Run Time System" ("Application:Kind")) -> (x = y?=w72:bool)
              n235 = case shown="True" w72 {
                tunnel: w73 -> [w74 w76]
                tunnel: [w74 w75] -> _
                frame False {
                }
                frame True {
                  n236 = invoke class="VI" method="FP.Close"(error in=w76) -> (error out=w75:errorcluster)  [unwired: 2 in, 2 out]
                }
              }
            }
          }
          n237 = while {
            stop <- w88 stop-if-true
            n238 = local read "Datalog directory path"() -> (w82:path)
            n239 = local read "Auto data log interval"() -> (w83:dbl)
            n240 = Multiply(x=i16 1000 ("y"), y=w83) -> (x*y=w85:dbl)
            n241 = call "auto datalogger.vi"("data log interval (s)"=w83, "Datalog directory path"=w82) -> ("File Failure"=→"Datalog File Failure":bool, "File refnum"=→"auto datalogref":refnum<file>)  [unwired: 8 in]
            n242 = Wait Until Next ms Multiple(millisecond multiple=w85) -> ()  [unwired: 1 out]
            n243 = local read "Quit"() -> (w88:bool)
          }
          n244 = while {
            stop <- w81 stop-if-true
            n245 = local read "user datalog ref"() -> (w78:refnum<file>)
            n246 = local read "User Data log interval"() -> (w77:dbl)
            n247 = call "auto datalogger user selected.vi"("data log interval (s)"=w77, "datalog ref"=w78) -> ()  [unwired: 8 in, 2 out]
            n248 = Multiply(x=i16 1000 ("y"), y=w77) -> (x*y=w79:dbl)
            n249 = local read "Quit"() -> (w81:bool)
            n250 = Wait Until Next ms Multiple(millisecond multiple=w79) -> ()  [unwired: 1 out]
          }
          n251 = while {
            shift-right: [w53] -> _
            shift-left: _ -> [w55]
            stop <- w58 stop-if-true
            n252 = call "share data state machine.vi"("Share data command"=share_data_command."Write data") -> ("Write data cluster out"=w54:T30)  [unwired: 4 in, 6 out]
            n253 = Unbundle By Name(w54) -> ("Data interval (s)"=w53:sgl)
            n254 = Multiply(x=i16 1000 ("y"), y=w55) -> (x*y=w57:sgl)
            n255 = local read "Quit"() -> (w58:bool)
            n256 = Wait Until Next ms Multiple(millisecond multiple=w57) -> ()  [unwired: 1 out]
          }
        }
      }
    }
  }
